vi "VariableManager_Variant.vi"(7 "Operation":enum16{"Get Tag", "Set Tag"}(ring), 8 "error in (no error)":errorcluster, 10 "Value":variant, 11 "Tag":string) -> (0 "error out":errorcluster, 2 "Value out":variant, 3 "Tag Out":string, 4 "Found":bool, 5 "All Tags":cluster{"Tags":string[], "Values":variant[]})   [LabVIEW 2018]
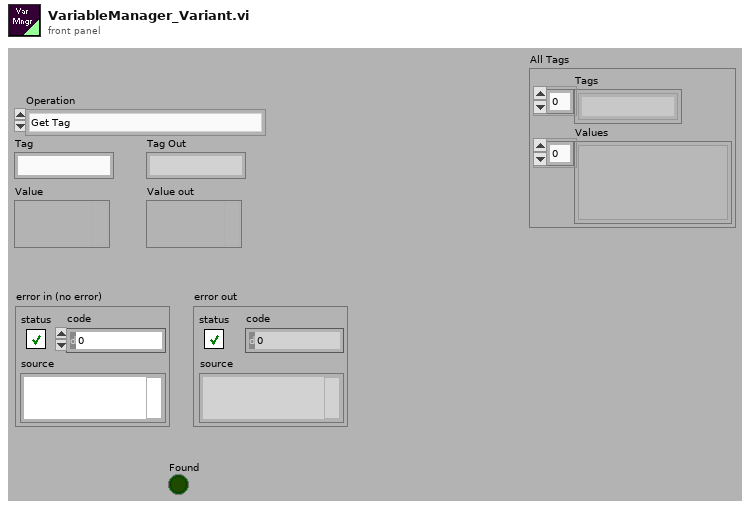
[diagram p1: front panel]
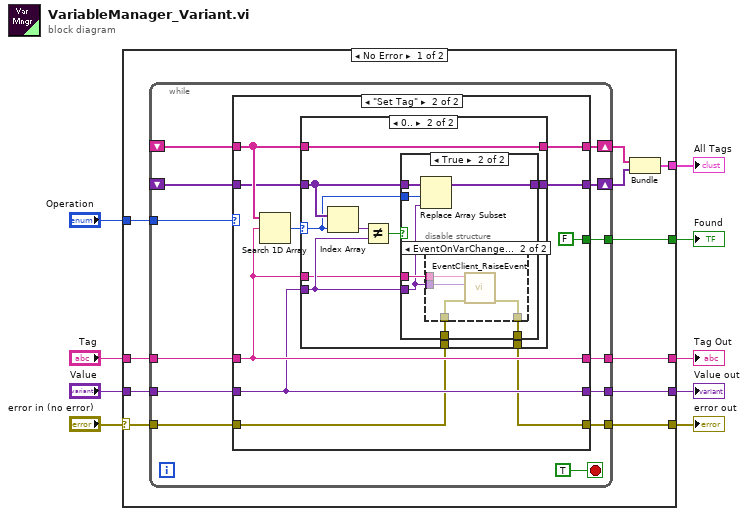
[diagram p0: block diagram]
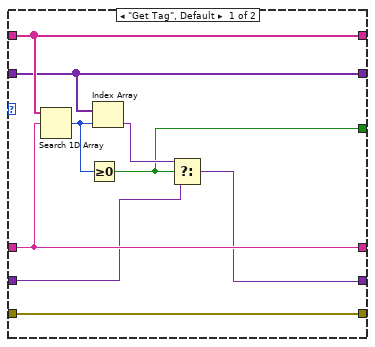
[diagram p2: hidden frame]
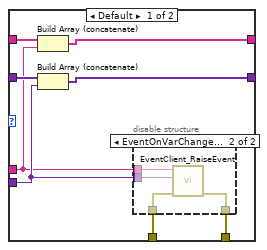
[diagram p3: hidden frame]
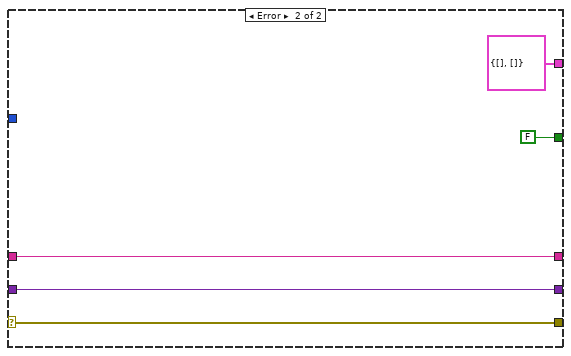
[diagram p7: hidden frame]
diagram:
  n1 = case shown="No Error" "error in (no error)" {
    selector: "error in (no error)" -> [w12 w92]
    tunnel: [w20 w94] -> w9
    tunnel: [w19 w93] -> w8
    tunnel: [w16 cluster{string[], variant[]} {[], []}] -> w7
    tunnel: [w15 w92] -> w6
    tunnel: "Tag" -> [w14 w94]
    tunnel: "Value" -> [w13 w93]
    tunnel: [w11 FALSE] -> w2
    tunnel: "Operation" -> [w10 _]
    frame No Error {
      n2 = while {
        shift-right: [w32] -> w18
        shift-left: _ -> [w33]
        shift-right: [w30] -> w17
        shift-left: _ -> [w31]
        tunnel: [w29] -> w20
        tunnel: [w28] -> w19
        tunnel: w12 -> [w26]
        tunnel: [w25] -> w15
        tunnel: w14 -> [w24]
        tunnel: w13 -> [w23]
        tunnel: [w22] -> w11
        tunnel: w10 -> [w21]
        stop <- TRUE stop-if-true
        n3 = case shown="\"Set Tag\"" w21 {
          tunnel: w33 -> [w42 w51]
          tunnel: [w42 w50] -> w32
          tunnel: w31 -> [w41 w48]
          tunnel: [w41 w49] -> w30
          tunnel: w24 -> [w40 w47]
          tunnel: w23 -> [w34 w46]
          tunnel: [w40 w47] -> w29
          tunnel: [w37 w46] -> w28
          tunnel: w26 -> [w36 w45]
          tunnel: [w36 w44] -> w25
          tunnel: [w35 FALSE] -> w22
          frame "Get Tag", Default {
            n4 = Search 1D Array(1D array=w42, element=w40) -> (index of element=w39:i32)  [unwired: 1 out]
            n5 = Greater Or Equal To 0?(x=w39) -> (x >= 0?=w35:bool)
            n6 = Index Array(array=w41, index=w39) -> (element=w38:variant)
            n7 = Select(t=w38, s=w35, f=w34) -> (s? t:f=w37:variant)
          }
          frame "Set Tag" {
            n8 = Search 1D Array(1D array=w51, element=w47) -> (index of element=w52:i32)  [unwired: 1 out]
            n9 = case shown="0.." w52 {
              selector: w52 -> [_ w70]
              tunnel: [w59 w75] -> w50
              tunnel: w51 -> [w60 w75]
              tunnel: [w57 w71] -> w49
              tunnel: w48 -> [w58 w72]
              tunnel: w47 -> [w55 w68]
              tunnel: w46 -> [w56 w69]
              tunnel: w45 -> [w54 w67]
              tunnel: [w53 w66] -> w44
              frame Default {
                n10 = Build Array (concatenate)(w60, w55) -> (w59:string[])
                n11 = Build Array (concatenate)(w58, w56) -> (w57:variant[])
                n12 = disable-structure shown="EventOnVarChange==True" {
                  disable-tunnel: w56 -> [_ w65]
                  disable-tunnel: w55 -> [_ w64]
                  disable-tunnel: w54 -> [w61 w63]
                  disable-tunnel: [w61 w62] -> w53
                  frame condition #0 (active) {
                  }
                  frame condition #1 {
                    n13 = call "EventClient_RaiseEvent.vi"("error in (no error)"=w63, "Data"=w65, "Event"=w64) -> ("error out"=w62:errorcluster)  [unwired: 1 in, 7 out]
                  }
                }
              }
              frame 0.. {
                n14 = Index Array(array=w72, index=w70) -> (element=w74:variant)
                n15 = Not Equal?(x=w74, y=w69) -> (x != y?=w73:bool)
                n16 = case shown="True" w73 {
                  tunnel: w72 -> [w77 w84]
                  tunnel: [w77 w83] -> w71
                  tunnel: w70 -> [_ w82]
                  tunnel: w69 -> [_ w78]
                  tunnel: w68 -> [_ w80]
                  tunnel: w67 -> [w76 w81]
                  tunnel: [w76 w79] -> w66
                  frame False {
                  }
                  frame True {
                    n17 = Replace Array Subset(array=w84, new element=w78, index=w82) -> (w83:variant[])
                    n18 = disable-structure shown="EventOnVarChange==True" {
                      disable-tunnel: w78 -> [_ w89]
                      disable-tunnel: w80 -> [_ w88]
                      disable-tunnel: w81 -> [w85 w87]
                      disable-tunnel: [w85 w86] -> w79
                      frame condition #0 (active) {
                      }
                      frame condition #1 {
                        n19 = call "EventClient_RaiseEvent.vi"("error in (no error)"=w87, "Data"=w89, "Event"=w88) -> ("error out"=w86:errorcluster)  [unwired: 1 in, 7 out]
                      }
                    }
                  }
                }
              }
            }
          }
        }
      }
      n20 = Bundle(w18, w17) -> (w16:cluster{string[], variant[]})  [unwired: 1 out]
    }
    frame Error {
    }
  }
  "Tag Out" <- w9
  "Value out" <- w8
  "All Tags" <- w7
  "error out" <- w6
  "Found" <- w2
